vi "ke37xx Initialize.vi"(0 "VISA resource name":refnum<visa-resource-name>="GPIB0::6::INSTR", 5 "ID Query? (T: Yes)":bool=TRUE, 7 "Reset? (T: Yes)":bool=TRUE, 11 "error in (no error)":errorcluster) -> (4 "VISA resource name out":refnum<visa-resource-name>, 15 "error out":errorcluster)   [LabVIEW 2009, in "Keithley 3700 Series.lvlib"]
doc: "This VI opens a VISA session for the VISA resource name specified. You can optionally reset the instrument by setting the front panel reset control. You must run this VI before using any of the instrument driver VIs for this instrument."
uses:
  <instrlib>/Keithley 3706/Keithley 3700 Series.lvlib
panel:
  # "© 2004 National Instruments Corporation.  ALL RIGHTS RESERVED."
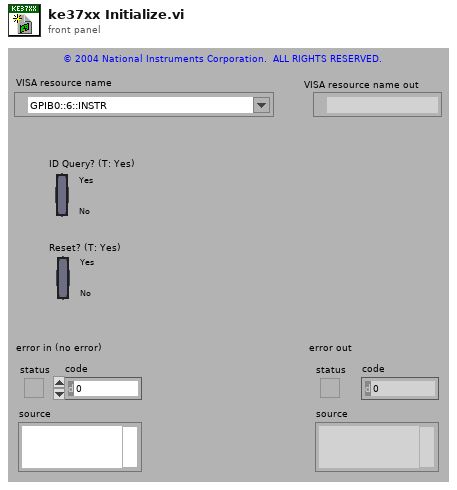
[diagram p1: front panel]
types:
  T1 = cluster{"Status":bool, "Code":i32, "Source (VI Name)":string}
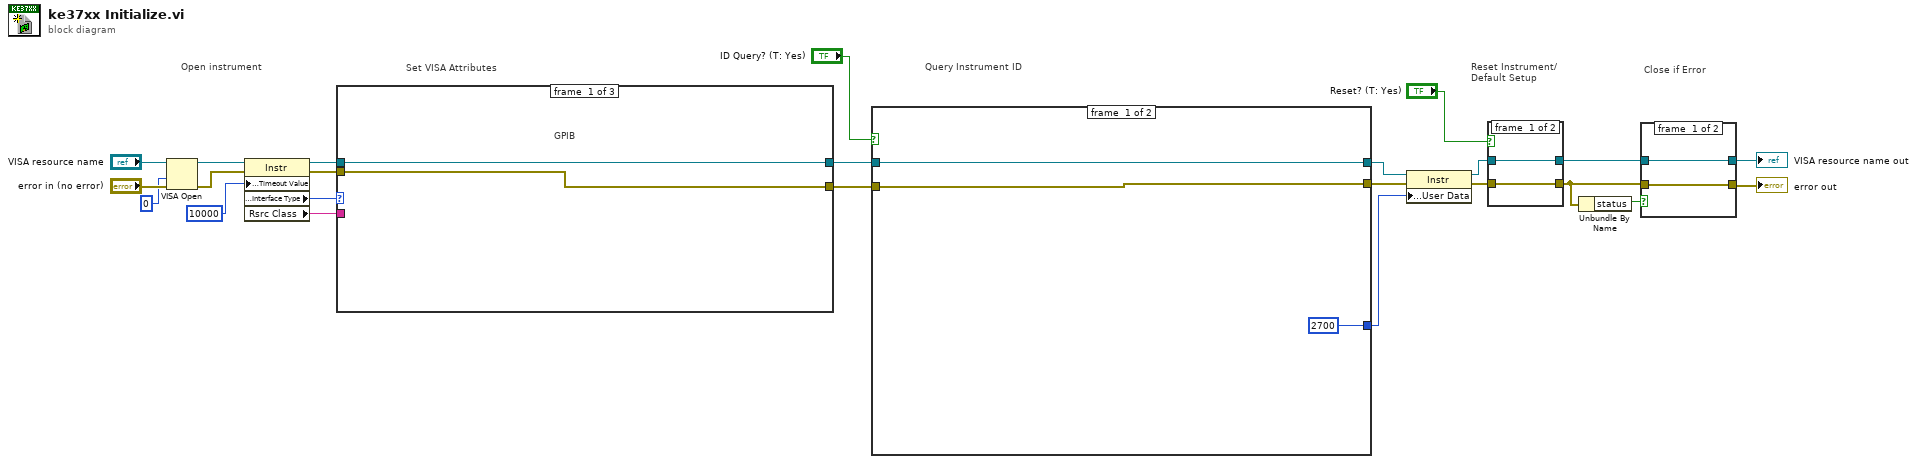
[diagram p0: block diagram]
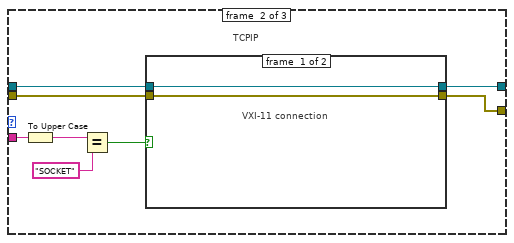
[diagram p2: hidden frame]
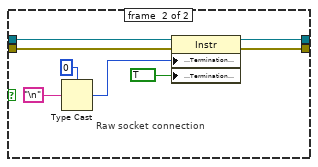
[diagram p3: hidden frame]
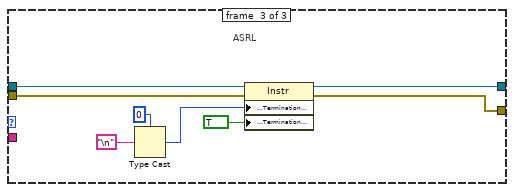
[diagram p4: hidden frame]
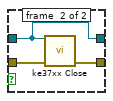
[diagram p5: hidden frame]
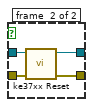
[diagram p6: hidden frame]
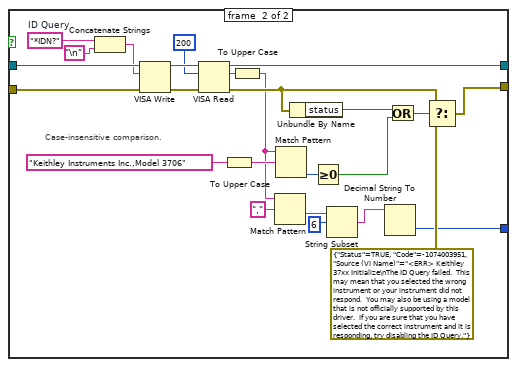
[diagram p7: hidden frame]
diagram:
  # "Set VISA Attributes"
  # "Close if Error"
  # "Query Instrument ID"
  # "Reset Instrument/\nDefault Setup"
  # "Open instrument"
  n1 = VISA Open(access mode=u32 0, error in (no error)="error in (no error)", VISA resource name="VISA resource name") -> (VISA resource name=w2:refnum<visa-resource-name>, error out=w3:errorcluster)  [unwired: 2 out]
  n2 = property class="Instr"(reference=w2, error in=w3, "General Settings:Timeout Value"=u32 10000) -> (reference out=w22:refnum<visa-resource-name>, error out=w23:errorcluster, "Interface Information:Interface Type"=w7:u16, "Rsrc Class"=w1:string)
  n3 = case shown="6" w7 {
    tunnel: [w25 w33 w51] -> w20
    tunnel: [w26 w32 w50] -> w21
    tunnel: w22 -> [w25 w31 w49]
    tunnel: w23 -> [w26 w34 w52]
    tunnel: w1 -> [_ w30 _]
    frame #0 {
      # "GPIB"
    }
    frame #1 {
      # "TCPIP"
      n4 = To Upper Case(1:w30) -> (0:w29:string)
      n5 = Equal?(x=w29, y="SOCKET" ("regular expression")) -> (x = y?=w27:bool)
      n6 = case shown="True" w27 {
        tunnel: w34 -> [w35 w44]
        tunnel: [w36 w43] -> w33
        tunnel: [w35 w42] -> w32
        tunnel: w31 -> [w36 w37]
        frame #0 {
          # "VXI-11 connection"
        }
        frame #1 {
          # "Raw socket connection"
          n7 = Type Cast(type=u8 0, x="\n") -> (*(type *) &x=w38:u8)
          n8 = property class="Instr"(reference=w37, error in=w44, "Message Based Settings:Termination Character"=w38, "Message Based Settings:Termination Character Enable"=TRUE) -> (reference out=w43:refnum<visa-resource-name>, error out=w42:errorcluster)
        }
      }
    }
    frame #2 {
      # "ASRL"
      n9 = Type Cast(type=u8 0, x="\n") -> (*(type *) &x=w45:u8)
      n10 = property class="Instr"(reference=w49, error in=w52, "Message Based Settings:Termination Character"=w45, "Message Based Settings:Termination Character Enable"=TRUE) -> (reference out=w51:refnum<visa-resource-name>, error out=w50:errorcluster)
    }
  }
  n11 = case shown="True" "ID Query? (T: Yes)" {
    tunnel: [w54 w80] -> w9
    tunnel: [w55 w70] -> w12
    tunnel: w20 -> [w55 w73]
    tunnel: w21 -> [w54 w74]
    tunnel: [2700 w63] -> w8
    frame #0 {
    }
    frame #1 {
      w62 = "*IDN?"  # ID Query
      # "Case-insensitive comparison."
      n12 = Concatenate Strings(w62, "\n") -> (w60:string)
      n13 = VISA Write(VISA resource name=w73, write buffer=w60, error in (no error)=w74) -> (VISA resource name out=w76:refnum<visa-resource-name>, error out=w75:errorcluster)  [unwired: 1 out]
      n14 = VISA Read(VISA resource name=w76, byte count=u32 200, error in (no error)=w75) -> (VISA resource name out=w70:refnum<visa-resource-name>, read buffer=w69:string, error out=w72:errorcluster)  [unwired: 1 out]
      n15 = To Upper Case(1:"Keithley Instruments Inc.,Model 3706") -> (0:w58:string)
      n16 = To Upper Case(1:w69) -> (0:w56:string)
      n17 = Match Pattern(string=w56, regular expression=",") -> (after substring=w66:string)  [unwired: 4 out]
      n18 = Match Pattern(string=w56, regular expression=w58) -> (offset past match=w67:i32)  [unwired: 4 out]
      n19 = Unbundle By Name(w72) -> ("status"=w78:bool)
      n20 = Greater Or Equal To 0?(x=w67) -> (x >= 0?=w59:bool)
      n21 = String Subset(string=w66, offset (0)=6) -> (substring=w64:string)  [unwired: 1 out]
      n22 = Decimal String To Number(string=w64) -> (number=w63:i32)  [unwired: 3 out]
      n23 = Or(x=w78, y=w59) -> (x .or. y?=w79:bool)
      n24 = Select(t=w72, s=w79, f=T1 {"Status"=TRUE, "Code"=-1074003951, "Source (VI Name)"="<ERR> Keithley 37xx Initialize\nThe ID Query failed.  This may mean that you selected the wrong instrument or your instrument did not respond.  You may also be using a model that is not officially supported by this driver.  If you are sure that you have selected the correct instrument and it is responding, try disabling the ID Query."}) -> (s? t:f=w80:T1)
    }
  }
  n25 = property on="Property Node" class="Instr"(reference=w12, error in=w9, "General Settings:User Data"=w8) -> (reference out=w11:refnum<visa-resource-name>, error out=w10:errorcluster)
  n26 = case shown="True" "Reset? (T: Yes)" {
    tunnel: w10 -> [w81 w85]
    tunnel: [w81 w84] -> w13
    tunnel: w11 -> [w82 w86]
    tunnel: [w82 w83] -> w14
    frame #0 {
    }
    frame #1 {
      n27 = call <instrlib>:"ke37xx Reset.vi"("VISA resource name"=w86, "error in (no error)"=w85) -> ("VISA resource name out"=w83:refnum<visa-resource-name>, "error out"=w84:errorcluster)  [unwired: 12 out]
    }
  }
  n28 = Unbundle By Name(w13) -> ("status"=w24:bool)
  n29 = case shown="True" w24 {
    tunnel: w14 -> [w88 w89]
    tunnel: [w88 w89] -> w6
    tunnel: [w87 w90] -> w5
    tunnel: w13 -> [w87 w91]
    frame #0 {
    }
    frame #1 {
      n30 = call <instrlib>:"ke37xx Close.vi"("VISA resource name"=w89, "error in (no error)"=w91) -> ("error out"=w90:errorcluster)  [unwired: 13 out]
    }
  }
  "VISA resource name out" <- w6
  "error out" <- w5
